vi "CALC_OFFS_MAGN.vi"(0 "VISA IN":refnum<visa-resource-name>, 1 "Offset Value(dB)":i32, 5 "error in":errorcluster, 7 "Channel":i32) -> (14 "VISA Out":refnum<visa-resource-name>, 19 "error out":errorcluster)   [LabVIEW 2018, in "PNA-X.lvlib"]
doc: "CALCulate<cnum>:OFFSet:MAGNitude <num>\n1550\n\n(Read-Write) Offsets the data trace magnitude by the specified value. \nTo offset the data trace magnitude to a slope value that changes with frequency, use \nCALC:OFFS:MAGN:SLOP \nSee Critical Note \nParameters \n<cnum> Channel number of the measurement. There must be a selected measurement \non that channel. If unspecified, <cnum> is set to 1. \n<num> Offset value in dB. \nExamples CALC:OFFS:MAGN:4 \ncalculate1:offset:magnitude -2 \nQuery Syntax CALCulate<cnum>:OFFSet:MAGNitude? \nReturn Type Numeric \nDefault 0"
uses:
  PNA-X.lvlib
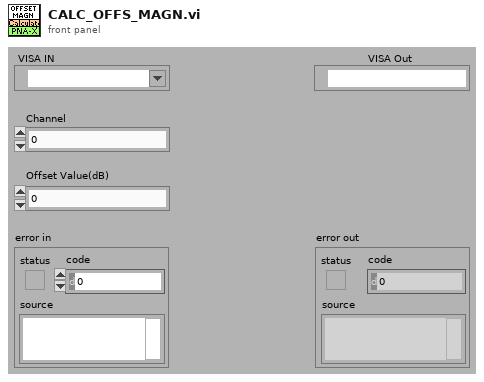
[diagram p1: front panel]
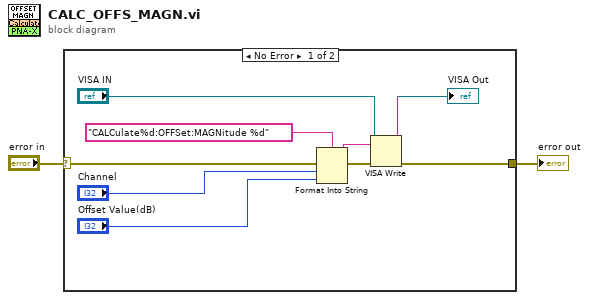
[diagram p0: block diagram]
diagram:
  n1 = case shown="No Error" "error in" {
    selector: "error in" -> [w11 w12]
    tunnel: [w6 w12] -> w1
    frame No Error {
      n2 = Format Into String(format string="CALCulate%d:OFFSet:MAGNitude %d" ("Cmdline"), error in=w11, "Channel", "Offset Value(dB)") -> (resulting string=w9:string, error out=w10:errorcluster)  [unwired: 1 in]
      n3 = VISA Write(VISA resource name="VISA IN", write buffer=w9, error in (no error)=w10) -> (VISA resource name out=→"VISA Out":refnum<visa-resource-name>, error out=w6:errorcluster)  [unwired: 1 out]
    }
    frame Error {
    }
  }
  "error out" <- w1
